vi "Create Queue MMain.vi"(8 "error in":errorcluster) -> (0 "error out":errorcluster, 3 "queMMain":refnum<queue>)   [LabVIEW 2014]
uses:
  Library/Queue/QueData.ctl
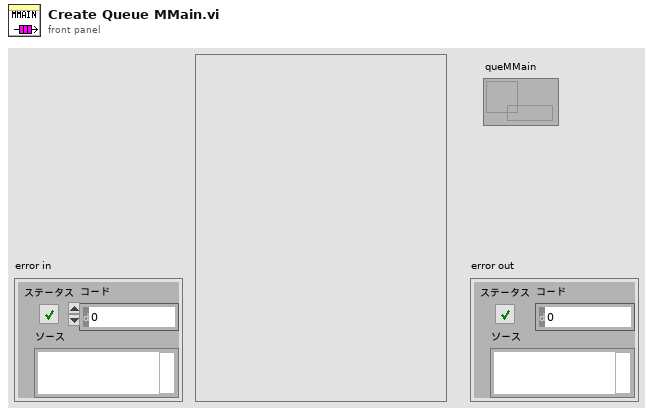
[diagram p1: front panel]
types:
  T1 = typedef "QueData.ctl" = cluster{"コマンド":string, "バリアント":variant}
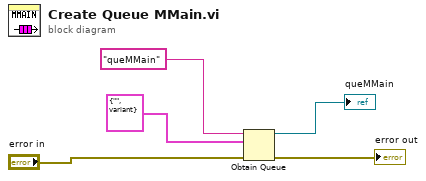
[diagram p0: block diagram]
diagram:
  n1 = Obtain Queue(name (unnamed)="queMMain" ("名前（名前なし）"), element data type=T1 {"コマンド"="", "バリアント"=variant}, error in (no error)="error in") -> (queue out=→"queMMain":refnum<queue>, error out=→"error out":errorcluster)  [unwired: 2 in, 1 out]
